vi "Read Cross Val.vi"(6 "Col Header Name 2":string, 7 "Section Name":string, 8 "error in (no error)":errorcluster, 9 "Col Header Val 1":string, 10 "Col Header Name 1":string, 11 "Config Data":T1(array[cluster])) -> (0 "error out":errorcluster, 1 "Col Header Val 2":string, 3 "Config Data dup":T1(array[cluster]), 4 "Key Find?":bool)   [LabVIEW 2020, in "GUCalibration2.lvlib"]
uses:
  GUCalibration2.lvlib
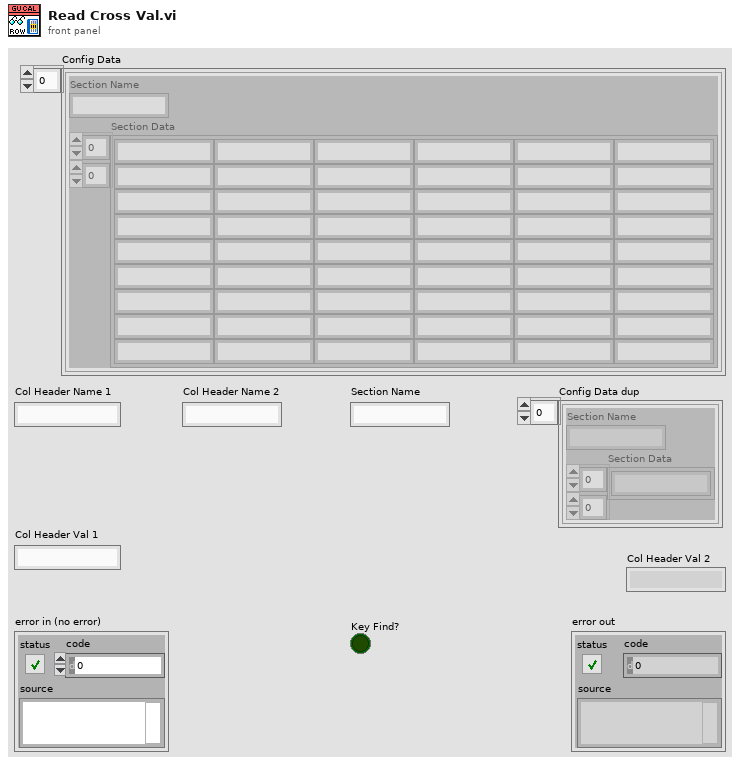
[diagram p1: front panel]
types:
  T1 = cluster{"Section Name":string, "Section Data":string[][]}[]
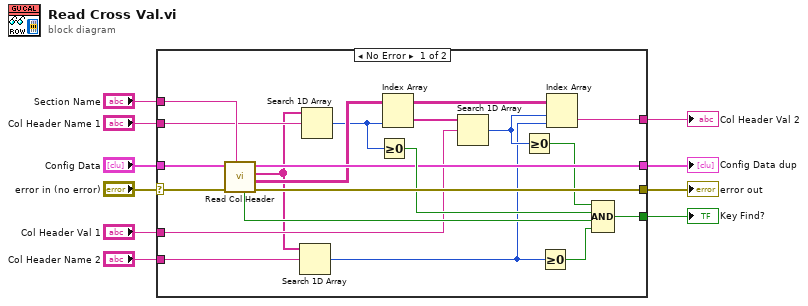
[diagram p0: block diagram]
diagram:
  n1 = case shown="No Error" "error in (no error)" {
    selector: "error in (no error)" -> [w28 w32]
    tunnel: "Section Name" -> [w29 _]
    tunnel: "Config Data" -> [w30 w31]
    tunnel: [w26 w32] -> w7
    tunnel: [w22 w31] -> w6
    tunnel: [w23 _] -> w5
    tunnel: [w15 _] -> w4
    tunnel: "Col Header Name 1" -> [w27 _]
    tunnel: "Col Header Val 1" -> [w20 _]
    tunnel: "Col Header Name 2" -> [w13 _]
    frame No Error {
      n2 = call "Read Col Header.vi"("Section Name"=w29, "error in (no error)"=w28, "Config Data"=w30) -> ("error out"=w26:errorcluster, "Data"=w18:string[][], "Column Header"=w14:string[], "Config Data dup"=w22:T1, "Section Find?"=w24:bool)  [unwired: 4 in]
      n3 = Search 1D Array(1D array=w14, element=w13) -> (index of element=w12:i32)  [unwired: 1 in]
      n4 = Search 1D Array(1D array=w14, element=w27) -> (index of element=w16:i32)  [unwired: 1 in]
      n5 = Greater Or Equal To 0?(x=w16) -> (x >= 0?=w25:bool)
      n6 = Index Array(array=w18, index (col)=w16) -> (element=w21:string[])  [unwired: 1 in]
      n7 = Search 1D Array(1D array=w21, element=w20) -> (index of element=w17:i32)  [unwired: 1 in]
      n8 = Greater Or Equal To 0?(x=w17) -> (x >= 0?=w19:bool)
      n9 = Greater Or Equal To 0?(x=w12) -> (x >= 0?=w11:bool)
      n10 = Index Array(array=w18, index (row)=w17, index (col)=w12) -> (element=w15:string)
      n11 = Compound Arithmetic op=AND(w19, w25, w24, w11) -> (w23:bool)
    }
    frame Error {
    }
  }
  "error out" <- w7
  "Col Header Val 2" <- w4
  "Config Data dup" <- w6
  "Key Find?" <- w5
